vi "Data handler-AOL Zstack.vi"(4 "Save image":bool, 5 "Save Ref image":bool, 6 "Single Frame Data":T2, 8 "error in (no error)":errorcluster, 9 "Live graph data queue in":T1, 10 "Logging queue element in":T5={"Imaging Protocol"=enum."Live Imaging", "Number of Trials"=0, "Frame Size"=512, "# Averaged frames"=0, "Dwell time (us)"=0.0, "Index of Z-plane"=0, "Timelapse?"=FALSE, "Logging process is active"=FALSE, "Speed logging enabled"=FALSE, "tdms file ref"=refnum, "path"=path "", "Trial Number"=0, "Expected # points acquired"=FALSE, "Manually stopped"=FALSE, "Last trial"=FALSE, "Ch0 data"=[], "Ch1 data"=[], "Ref Data"=[], "Ref Frame Time"=[], "Image Time"=[], "Continuous Time"=[], "Ref X Length"=0, "Ref Y Length"=0, "# Ref Averaged frames"=0, "Ref Dwell time (us)"=0.0, "Points acquired"={"Ch0 last trial"=0, "Ch1 last trial"=0, "All trials"=0}, "HW Timings File"=refnum} {"Ref Dwell time (us)" format="%#.6g"; "Frame Size" items=["100X100"=100, "128X128"=128, "200X200"=200, "256X256"=256, "512X512"=512, "1024x1024"=1024, "2048x2048"=2048]; "Dwell time (us)" format="%#.6g"}, 11 "Image array":T3) -> (0 "error out":errorcluster)   [LabVIEW 2020]
uses:
  Typedefs/Logging queue element.ctl
  Typedefs/Imaging Protocols enum.ctl
  Typedefs/Frame Size.ctl
  Typedefs/Acquired points count.ctl
  User Interface/Queue/Live graphs queue/Typedefs/Live imaging queue element.ctl
  <vilib>/vision/Image Controls.llb/IMAQ Image.ctl
  Typedefs/Frame data dual cluster.ctl
  User Interface/Typedefs/Live graph data queue ref.ctl
  Typedefs/Subpanel close request.ctl
  Typedefs/Top level VI states.ctl
  Typedefs/Channel Selector.ctl
  Global Variables/General Globals.vi
panel:
  out "Subpanel is closed / Proceed":bool
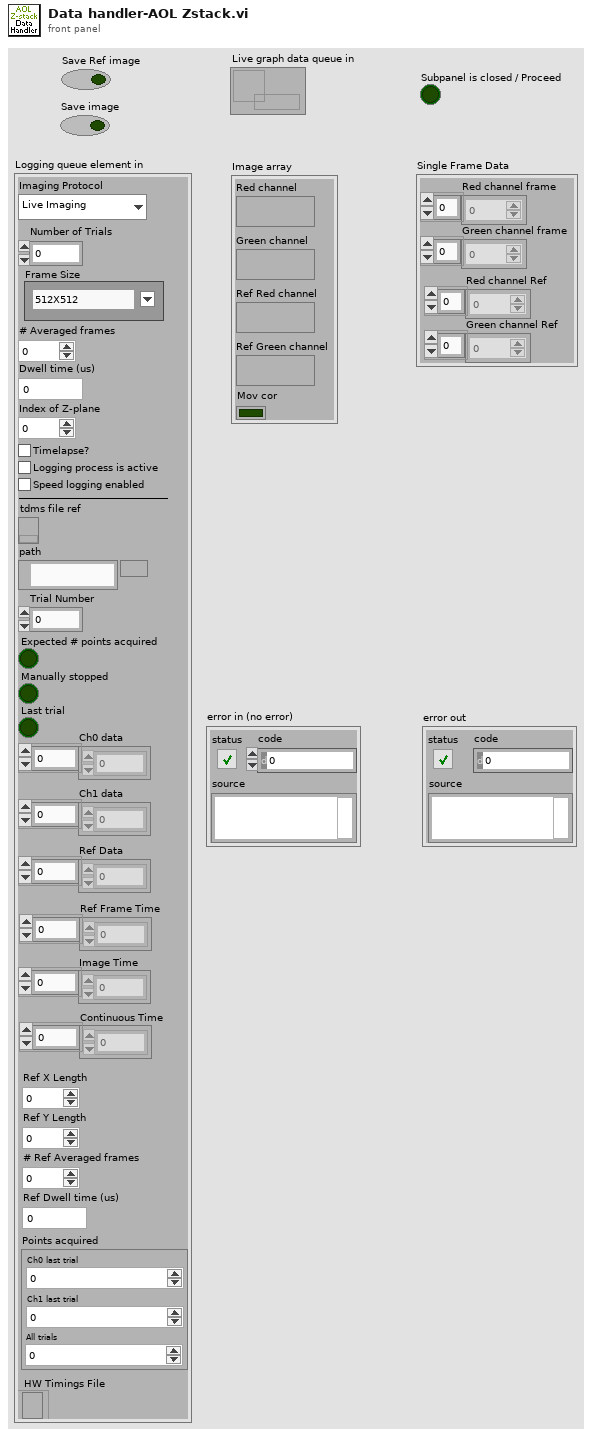
[diagram p1: front panel]
types:
  T1 = typedef "Live graph data queue ref.ctl" = refnum<queue>
  T2 = typedef "Frame data dual cluster.ctl" = cluster{"Red channel frame":dbl[], "Green channel frame":dbl[], "Red channel Ref":dbl[], "Green channel Ref":dbl[]}
  T3 = typedef "Live imaging queue element.ctl" = cluster{"Red channel":T4, "Green channel":T4, "Ref Red channel":T4, "Ref Green channel":T4, "Mov cor":bool}
  T4 = typedef "IMAQ Image.ctl" = refnum<image>
  T5 = typedef "Logging queue element.ctl" = cluster{"Imaging Protocol":T6, "Number of Trials":u16, "Frame Size":T7, "# Averaged frames":u16, "Dwell time (us)":dbl, "Index of Z-plane":i32, "Timelapse?":bool, "Logging process is active":bool, "Speed logging enabled":bool, "tdms file ref":refnum<k34>, "path":path, "Trial Number":i32, "Expected # points acquired":bool, "Manually stopped":bool, "Last trial":bool, "Ch0 data":u32[], "Ch1 data":u32[], "Ref Data":u32[], "Ref Frame Time":u64[], "Image Time":u64[], "Continuous Time":u64[], "Ref X Length":u16, "Ref Y Length":u16, "# Ref Averaged frames":u16, "Ref Dwell time (us)":dbl, "Points acquired":T8, "HW Timings File":refnum<file>}
  T6 = typedef "Imaging Protocols enum.ctl" = enum16{"AOL Z-Stack", "Motor Z Stack", "Functional Acquisition", "Single Plane Acquisition", "Volume Acquisition", "Live Imaging", "Live Plane Imaging", "Live Volume Imaging"}
  T7 = typedef "Frame Size.ctl" = u16
  T8 = typedef "Acquired points count.ctl" = cluster{"Ch0 last trial":u64, "Ch1 last trial":u64, "All trials":u64}
  T9 = typedef "Subpanel close request.ctl" = enum16{"Request subpanel close", "Just check subpanel is closed"}
  T10 = typedef "Top level VI states.ctl" = enum16{"None", "Initialise UI", "<STACK PROTOCOL STATES>", "AOL Zstack-START", "AOL Zstack-STOP", "Motor Zstack-START", "Motor Zstack-STOP", "<ACQUISITION PROTOCOL STATES> ", "Functional Acquisition-START", "Functional Acquisition-STOP", "Single Plane Acquisition-START", "Single Plane Acquisition-STOP", "Volume Acquisition-START", "Volume Acquisition-STOP", "<LIVE IMAGING PROTOCOL STATES>", "Live Imaging-START", "Live Imaging-STOP", "Live Plane Imaging-START", "Live Plane Imaging-STOP", "Live Volume Imaging-START", "Live Volume Imaging-STOP", "<MOVEMENT CORRECTION PROTOCOL STATES>", "EXIT"}
  T11 = enum16{"open", "replace", "create", "open or create", "replace or create", "replace or create with confirmation"}
  T12 = typedef "Channel Selector.ctl" = enum16{"Red Channel", "Green Channel", "Blended"}
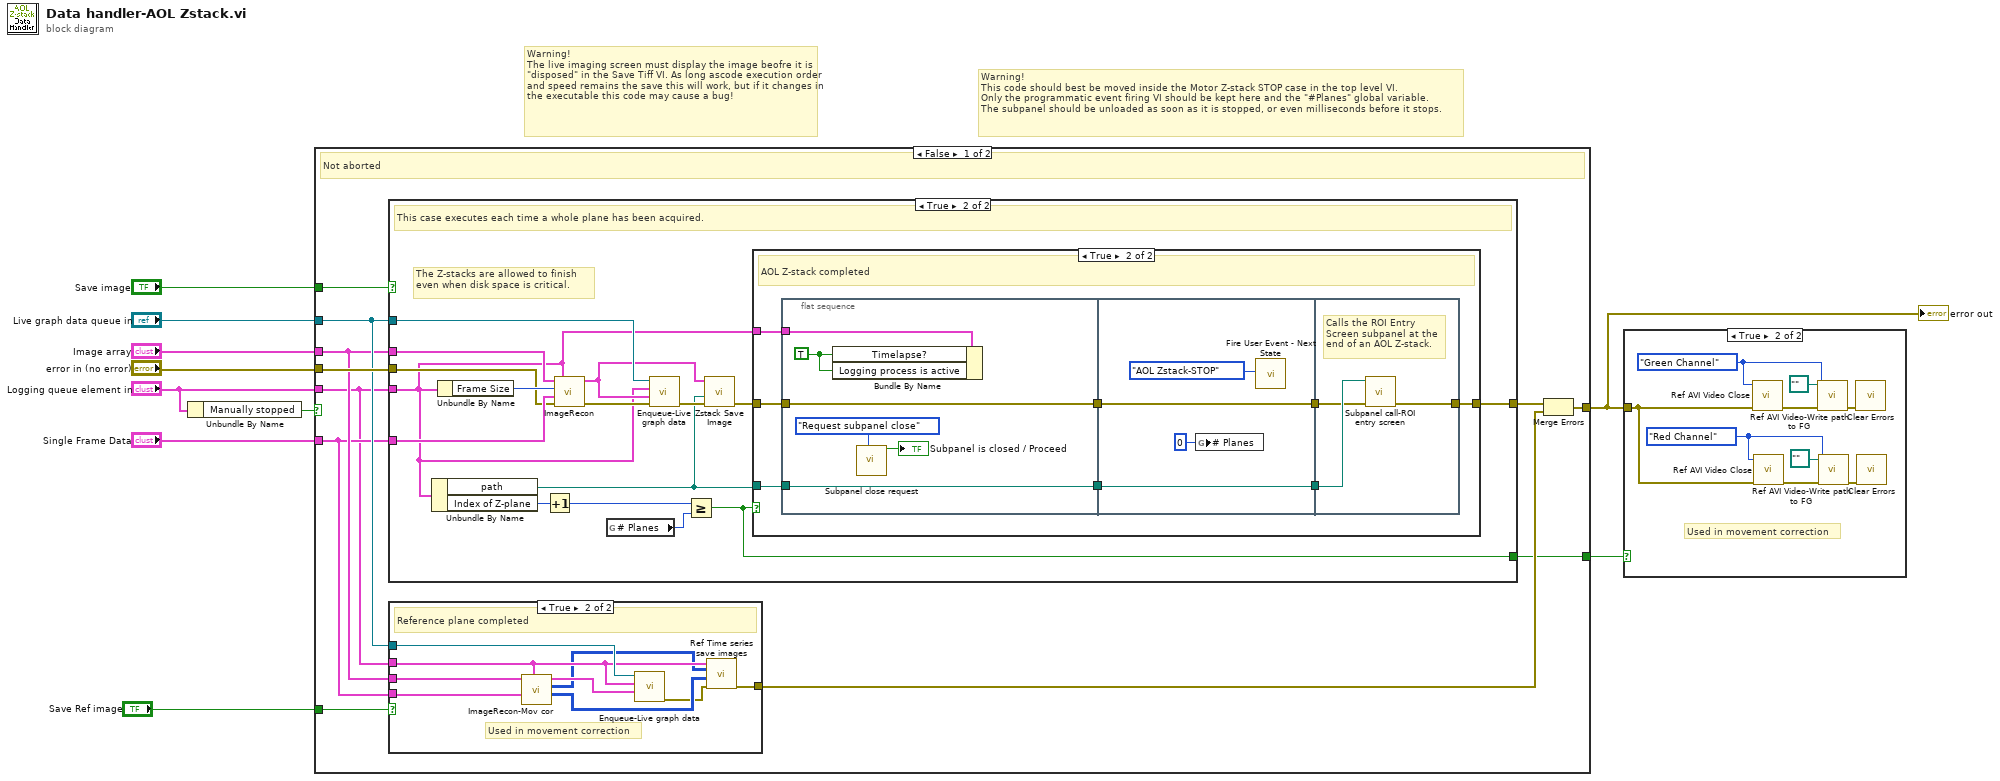
[diagram p0: block diagram]
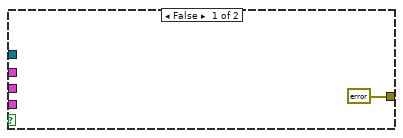
[diagram p2: hidden frame]
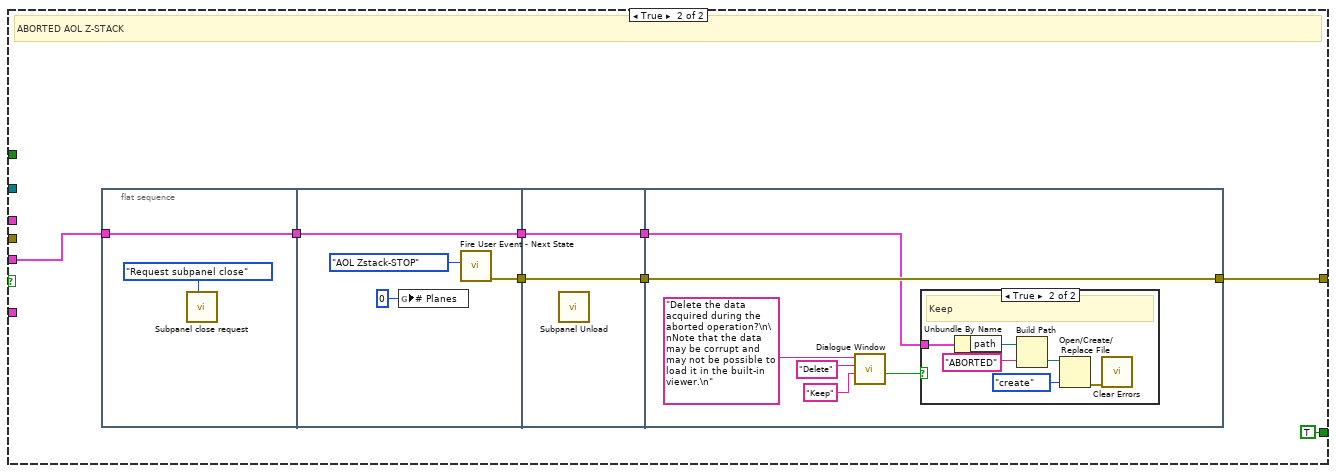
[diagram p5: hidden frame]
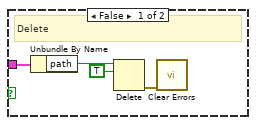
[diagram p6: hidden frame]
diagram:
  # "Warning!\nThe live imaging screen must display the image beofre it is \"disposed\" in the Save Tiff VI. As long ascode execution order and speed remains the save this will work, but if it changes in the executable this code may cause a bug!"
  # "Warning!\nThis code should best be moved inside the Motor Z-stack STOP case in the top level VI.\nOnly the programmatic event firing VI should be kept here and the \"#Planes\" global variable.\nThe subpanel should be unloaded as soon as it is stopped, or even milliseconds before it stops."
  n1 = Unbundle By Name("Logging queue element in") -> ("Manually stopped"=w1:bool)
  n2 = case shown="False" w1 {
    tunnel: "Save image" -> [w20 _]
    tunnel: "error in (no error)" -> [w19 _]
    tunnel: "Live graph data queue in" -> [w18 _]
    tunnel: "Image array" -> [w17 _]
    tunnel: "Single Frame Data" -> [w16 _]
    tunnel: [w14 w76] -> w5
    tunnel: "Save Ref image" -> [w13 _]
    tunnel: [w12 TRUE] -> w3
    tunnel: "Logging queue element in" -> [w11 w73]
    frame False {
      # "Not aborted"
      n3 = case shown="True" w20 {
        tunnel: [_ w47] -> w21
        tunnel: w17 -> [_ w45]
        tunnel: w11 -> [_ w33]
        tunnel: w16 -> [_ w42]
        tunnel: w19 -> [_ w41]
        tunnel: w18 -> [_ w40]
        tunnel: [_ w32] -> w12
        frame False {
          # "Acquisition of the current plane has not completed. Plane is incomplete."
        }
        frame True {
          # "The Z-stacks are allowed to finish even when disk space is critical."
          # "This case executes each time a whole plane has been acquired."
          n4 = Unbundle By Name(w33) -> ("path"=w37:path, "Index of Z-plane"=w43:i32)
          n5 = Unbundle By Name(w33) -> ("Frame Size"=w44:T7)
          n6 = Increment(x=w43) -> (x+1=w46:i32)
          n7 = call "ImageRecon.vi"("Logging queue element in"=w33, "Error In"=w41, "Data"=w42, "Frame Size"=w44, "Image Array (in)"=w45) -> ("Error Out"=w36:errorcluster, "Image Array(out)"=w35:T3)  [unwired: 3 in, 2 out]
          n8 = global read "General Globals.vi" "# Planes"() -> (w34:i32)
          n9 = call "Enqueue-Live graph data.vi"("error in (no error)"=w36, "Element to queue"=w35, "Logging queue element"=w33, "Live graph data queue in"=w40) -> ("error out"=w39:errorcluster)  [unwired: 6 in, 1 out]
          n10 = Greater Or Equal?(x=w46, y=w34) -> (x >= y?=w32:bool)
          n11 = call "Zstack Save Image.vi"("error in (no error)"=w39, "Dataset base-path"=w37, "Image Array"=w35) -> ("error out"=w38:errorcluster)  [unwired: 8 in]
          n12 = case shown="True" w32 {
            tunnel: w38 -> [w48 w54]
            tunnel: w37 -> [_ w56]
            tunnel: [w48 w55] -> w47
            tunnel: w33 -> [_ w49]
            frame False {
            }
            frame True {
              # "AOL Z-stack completed"
              n13 = flat-sequence {
                tunnel: w54 -> [w61]
                tunnel: w56 -> [w62]
                tunnel: [w62] -> w51
                tunnel: [w61] -> w50
                tunnel: w49 -> [w60]
                tunnel: [w66] -> w53
                tunnel: [w63] -> w52
                tunnel: w51 -> [w66]
                tunnel: w50 -> [w63]
                tunnel: [w68] -> w55
                tunnel: w53 -> [w69]
                tunnel: w52 -> [w67]
                frame #0 {
                  w59 = TRUE ("Timelapse?")
                  n14 = Bundle By Name(cluster=w60, "Timelapse?"=w59, "Logging process is active"=w59) -> ()  [unwired: 1 out]
                  n15 = call "Subpanel close request.vi"("Function"=Subpanel_close_request."Request subpanel close") -> ("Subpanel is closed / Proceed"=→"Subpanel is closed / Proceed":bool)  [unwired: 10 in]
                }
                frame #1 {
                  n16 = global write "General Globals.vi" "# Planes"(0 ("# Planes")) -> ()
                  n17 = call "Fire User Event - Next State.vi"("\"UI Handler loop\" case to execute"=Top_level_VI_states."AOL Zstack-STOP" ("event data / imaging mode")) -> ()  [unwired: 10 in, 1 out]
                }
                frame #2 {
                  # "Calls the ROI Entry Screen subpanel at the end of an AOL Z-stack."
                  n18 = call "Subpanel call-ROI entry screen.vi"("error in"=w67, "Experiment folder path"=w69) -> ("error out"=w68:errorcluster)  [unwired: 9 in]
                }
              }
            }
          }
        }
      }
      n19 = case shown="True" w13 {
        tunnel: w11 -> [_ w28]
        tunnel: [errorcluster {"status"=FALSE, "code"=0, "source"=""} ("error out") w31] -> w15
        tunnel: w18 -> [_ w30]
        tunnel: w17 -> [_ w29]
        tunnel: w16 -> [_ w26]
        frame False {
        }
        frame True {
          # "Used in movement correction"
          # "Reference plane completed"
          n20 = call "ImageRecon-Mov cor.vi"("Logging queue element in"=w28, "Data"=w26, "Image Array (in)"=w29) -> ("Ch1-Green-REF"=w24:i16[][], "Ch0-Red-REF"=w25:i16[][], "Image Array(out)"=w27:T3)  [unwired: 5 in, 1 out]
          n21 = call "Enqueue-Live graph data.vi"("Element to queue"=w27, "Logging queue element"=w28, "Live graph data queue in"=w30) -> ("error out"=w23:errorcluster)  [unwired: 7 in, 1 out]
          n22 = call "Ref Time series save images.vi"("error in (no error)"=w23, "Ch1-Green-REF"=w24, "Ch0-Red-REF"=w25, "Logging queue element"=w28) -> ("error"=w31:errorcluster)  [unwired: 7 in]
        }
      }
      n23 = Merge Errors(w21, w15) -> (w14:errorcluster)
    }
    frame True {
      # "ABORTED AOL Z-STACK"
      n24 = flat-sequence {
        tunnel: w73 -> [w78]
        tunnel: [w78] -> w72
        tunnel: [w81] -> w75
        tunnel: w72 -> [w80]
        tunnel: [w80] -> w71
        tunnel: w75 -> [w85]
        tunnel: [w85] -> w74
        tunnel: w71 -> [w84]
        tunnel: [w84] -> w70
        tunnel: [w91] -> w76
        tunnel: w74 -> [w91]
        tunnel: w70 -> [w87]
        frame #0 {
          n25 = call "Subpanel close request.vi"("Function"=Subpanel_close_request."Request subpanel close") -> ()  [unwired: 10 in, 1 out]
        }
        frame #1 {
          n26 = global write "General Globals.vi" "# Planes"(0 ("# Planes")) -> ()
          n27 = call "Fire User Event - Next State.vi"("\"UI Handler loop\" case to execute"=Top_level_VI_states."AOL Zstack-STOP" ("event data / imaging mode")) -> ("Error Out"=w81:errorcluster)  [unwired: 10 in]
        }
        frame #2 {
          n28 = call "Subpanel Unload.vi"() -> ()  [unwired: 11 in, 1 out]
        }
        frame #3 {
          n29 = call "Dialogue Window.vi"("Caption-Left button (Cancel)"="Keep", "Caption-Right button (OK)"="Delete", "Message string"="Delete the data acquired during the aborted operation?\n\nNote that the data may be corrupt and may not be possible to load it in the built-in viewer.\n") -> ("Cancelled (Left button pressed)"=w88:bool)  [unwired: 6 in, 2 out]
          n30 = case shown="True" w88 {
            tunnel: w87 -> [w95 w96]
            frame False {
              # "Delete"
              n31 = Unbundle By Name(w95) -> ("path"=w94:path)
              n32 = Delete(path (use dialog)=w94, entire hierarchy (F)=TRUE) -> (error out=w92:errorcluster)  [unwired: 3 in, 2 out]
              n33 = call <vilib>:"Clear Errors.vi"("error in (no error)"=w92) -> ()  [unwired: 5 in, 2 out]
            }
            frame True {
              # "Keep"
              n34 = Unbundle By Name(w96) -> ("path"=w101:path)
              n35 = Build Path(base path=w101, name or relative path="ABORTED") -> (appended path=w98:path)
              n36 = Open/Create/Replace File(file path (use dialog)=w98, operation (0:open)=T11."create") -> (error out=w100:errorcluster)  [unwired: 4 in, 2 out]
              n37 = call <vilib>:"Clear Errors.vi"("error in (no error)"=w100) -> ()  [unwired: 5 in, 2 out]
            }
          }
        }
      }
    }
  }
  "error out" <- w5
  n38 = case shown="True" w3 {
    tunnel: w5 -> [_ w104]
    frame False {
    }
    frame True {
      w102 = Channel_Selector."Red Channel" ("Channel")
      w103 = Channel_Selector."Green Channel" ("Channel")
      # "Used in movement correction"
      n39 = call "Ref AVI Video Close.vi"("error in (no error)"=w104, "Channel"=w103) -> ("error out"=w110:errorcluster)  [unwired: 9 in]
      n40 = call "Ref AVI Video Close.vi"("error in (no error)"=w104, "Channel"=w102) -> ("error out"=w105:errorcluster)  [unwired: 9 in]
      n41 = call "Ref AVI Video-Write path to FG.vi"("error in (no error)"=w110, "Channel"=w103, "AVI2 path"=path "") -> ("error out"=w108:errorcluster)  [unwired: 8 in]
      n42 = call "Ref AVI Video-Write path to FG.vi"("error in (no error)"=w105, "Channel"=w102, "AVI2 path"=path "") -> ("error out"=w107:errorcluster)  [unwired: 8 in]
      n43 = call <vilib>:"Clear Errors.vi"("error in (no error)"=w108) -> ()  [unwired: 5 in, 2 out]
      n44 = call <vilib>:"Clear Errors.vi"("error in (no error)"=w107) -> ()  [unwired: 5 in, 2 out]
    }
  }
